vi "Linespread_Function.vi"(8 "error in (no error)":errorcluster, 9 "Paramter guess":dbl[](array[numeric])=[165.0, 0.2, 0.1], 10 "y":dbl[](array[numeric]), 11 "x":dbl[](array[numeric])) -> (0 "error out":errorcluster, 2 "XY Graph":cluster{cdb[]}[](graph), 3 "best fit parameters":dbl[](array[numeric]))   [LabVIEW 2012, in "DAQOrcaFlash.lvclass"]
uses:
  DAQOrcaFlash.lvclass
  <vilib>/gmath/NumericalOptimization/Nonlinear Curve Fit LM.vi
  <vilib>/gmath/NI_Gmath.lvlib
panel:
  # "y min"
  # "y mean"
  # "A"
  # "STD"
  # "x0"
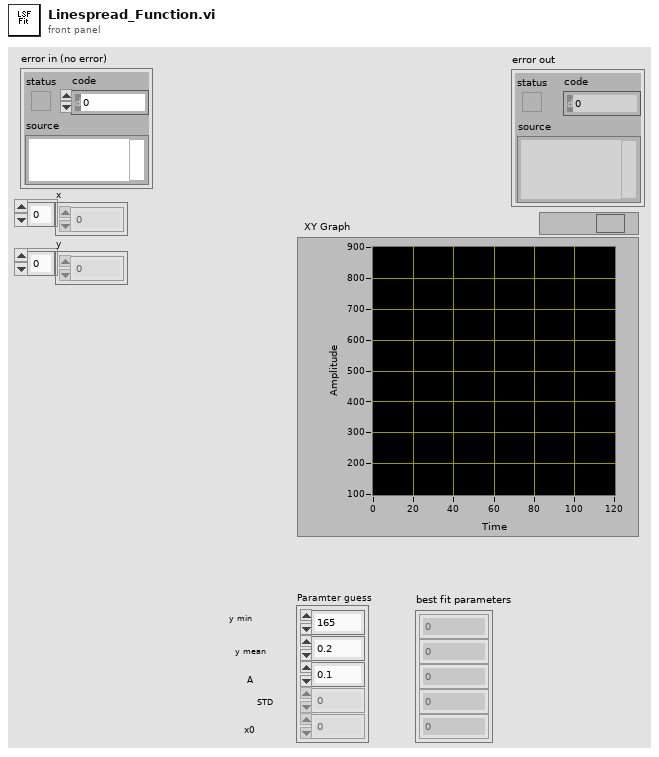
[diagram p1: front panel]
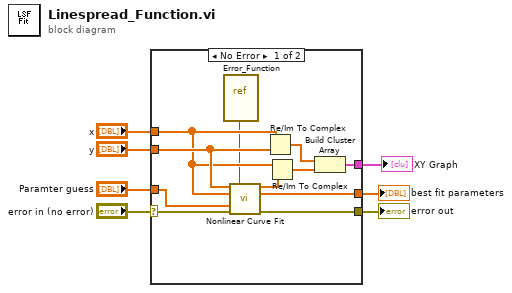
[diagram p0: block diagram]
diagram:
  n1 = case shown="No Error" "error in (no error)" {
    selector: "error in (no error)" -> [w8 w19]
    tunnel: [w16 _] -> w6
    tunnel: "y" -> [w15 _]
    tunnel: "x" -> [w14 _]
    tunnel: "Paramter guess" -> [w13 _]
    tunnel: [w11 w19] -> w5
    tunnel: [w9 _] -> w3
    frame No Error {
      n2 = vi-ref "Error_Function.vi"() -> (w12:refnum<vi>)
      n3 = call-poly <vilib>:"Nonlinear Curve Fit.vi"("Y"=w15, "f(x,a)"=w12, "X"=w14, "initial parameters"=w13, "error in (no error)"=w8) -> ("best nonlinear fit"=w10:dbl[], "best fit parameters"=w9:dbl[], "error out"=w11:errorcluster)  [unwired: 5 in, 3 out]
      n4 = Re/Im To Complex(1:w15, 2:w14) -> (0:w18:cdb[])
      n5 = Re/Im To Complex(1:w10, 2:w14) -> (0:w17:cdb[])
      n6 = Build Cluster Array(w18, w17) -> (w16:cluster{cdb[]}[])
    }
    frame Error {
    }
  }
  "XY Graph" <- w6
  "error out" <- w5
  "best fit parameters" <- w3
